vi "prepractica 4.vi"() -> ()   [LabVIEW 2015]
panel:
  in  "Clave":string
  out "Error":bool
  out "Comprobando:":string
  out "Correcto":bool
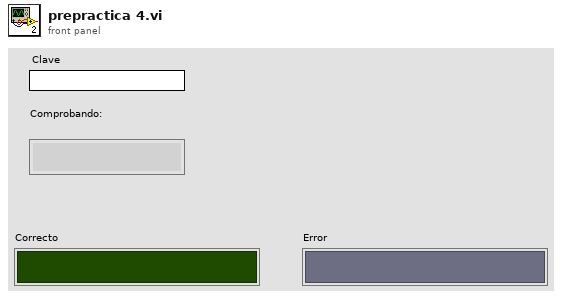
[diagram p1: front panel]
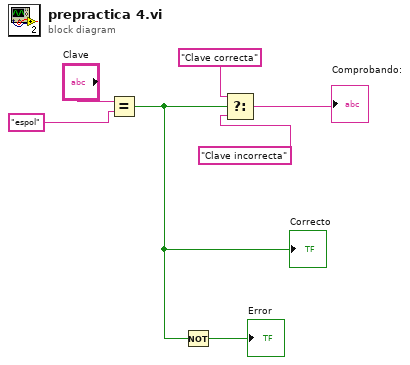
[diagram p0: block diagram]
diagram:
  n1 = Equal?(x="Clave", y="espol") -> (x = y?=w2:bool)
  "Correcto" <- w2
  n2 = Not(x=w2) -> (.not. x?=→"Error":bool)
  n3 = Select(t="Clave correcta", s=w2, f="Clave incorrecta") -> (s? t:f=→"Comprobando:":string)
